vi "DMSC.manage_process.vi"(0 "Process":T1 {"restartMode" items=["UNKNOWN", "MANUAL", "ONCE", "ALWAYS", "KILL", "SHUTDOWN"]}, 1 "procNames":string[](array[string]), 2 "procID":i32[](array[numeric]), 3 "procMemory":i32[](array[numeric]), 4 "procRuntime":dbl[](array[numeric]), 5 "SDConnectionEvent":refnum<user-event>) -> (14 "Process (out)":T1 {"restartMode" items=["UNKNOWN", "MANUAL", "ONCE", "ALWAYS", "KILL", "SHUTDOWN"]})   [LabVIEW 2014, in "DMSClient.lvlib"]
doc: "Manages (start/kill) processes"
uses:
  DMSClient.lvlib
  DMSC.process_type.ctl
  DomainManagementUtils/DMSU.restart_mode.ctl
  DomainManagementUtils/DMSUtils.lvlib
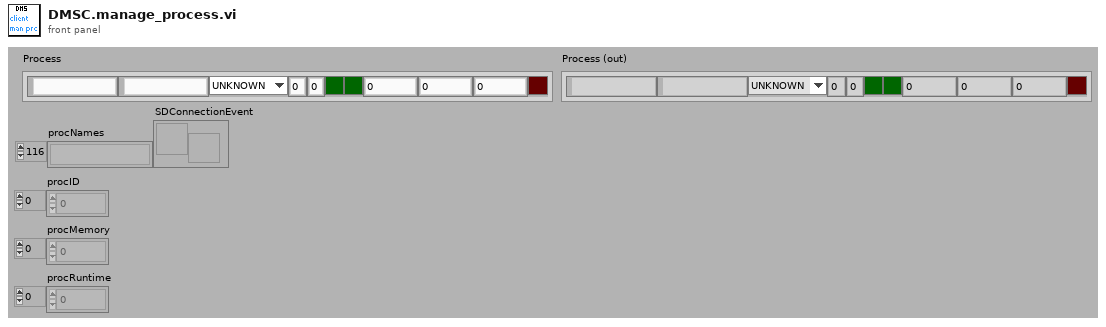
[diagram p1: front panel]
types:
  T1 = typedef "DMSClient.lvlib/DMSC.process_type.ctl" = cluster{"imageName":string, "argumentString":string, "restartMode":T2, "nOfRestart":i32, "resetRestartTimer":i32, "killOnExit":bool, "csSystem":bool, "PID":dbl, "PMem":dbl, "CPUTime":dbl, "startCnt":i32, "startTime":u32, "restartFailed":bool}
  T2 = typedef "DMSUtils.lvlib/DMSU.restart_mode.ctl" = u16
  T3 = cluster{"Command":enum16{"NewSystem", "DestroySystem", "SDSystem"}, "argumentString":string}
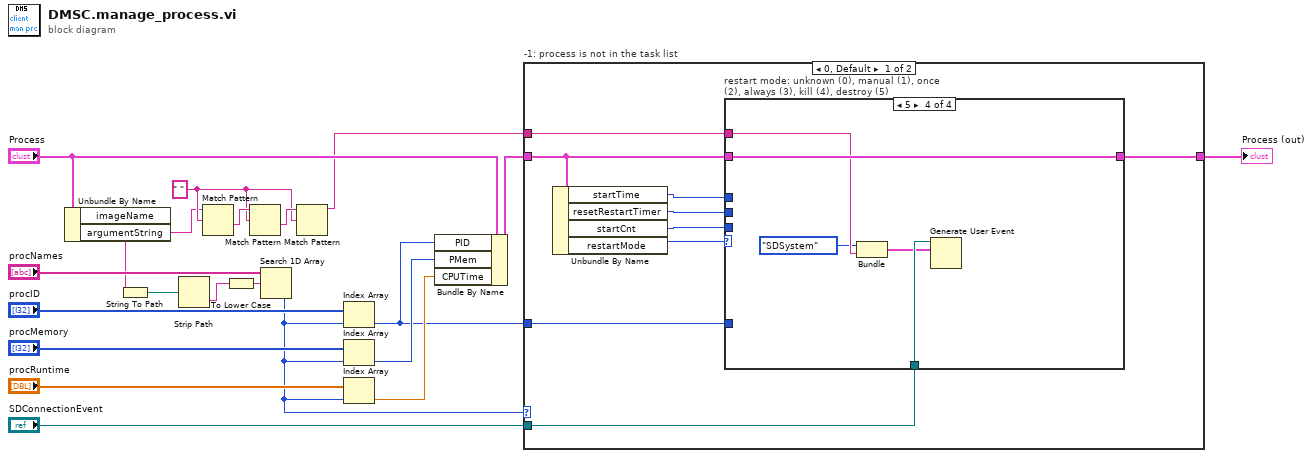
[diagram p0: block diagram]
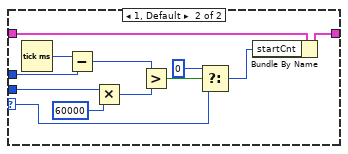
[diagram p3: hidden frame]
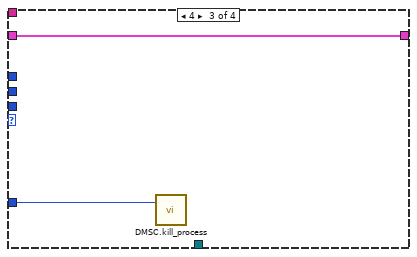
[diagram p5: hidden frame]
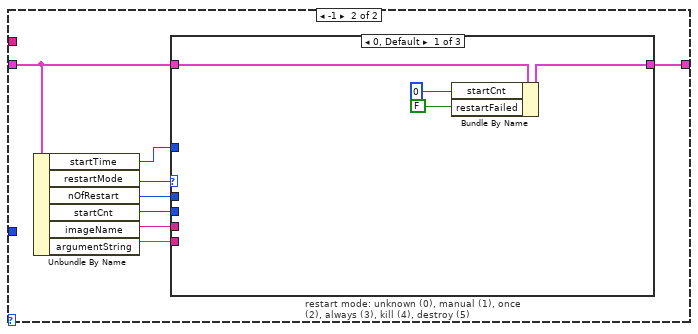
[diagram p6: hidden frame]
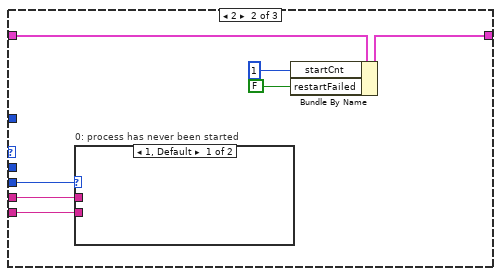
[diagram p7: hidden frame]
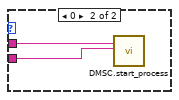
[diagram p8: hidden frame]
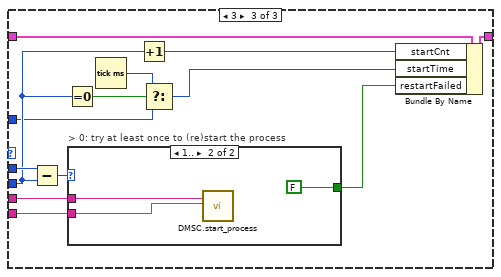
[diagram p9: hidden frame]
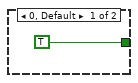
[diagram p10: hidden frame]
diagram:
  w4 = " " ("regular expression")
  n1 = Unbundle By Name("Process") -> ("imageName"=w8:string, "argumentString"=w3:string)
  n2 = String To Path(string=w8) -> (path=w9:path)
  n3 = Strip Path(path=w9) -> (name=w7:string)  [unwired: 1 out]
  n4 = Match Pattern(string=w3, regular expression=w4) -> (after substring=w6:string)  [unwired: 1 in, 3 out]
  n5 = To Lower Case(string=w7) -> (all lower case string=w10:string)
  n6 = Match Pattern(string=w6, regular expression=w4) -> (after substring=w5:string)  [unwired: 1 in, 3 out]
  n7 = Search 1D Array(1D array="procNames", element=w10) -> (index of element=w14:i32)  [unwired: 1 in]
  n8 = Match Pattern(string=w5, regular expression=w4) -> (before substring=w2:string)  [unwired: 1 in, 3 out]
  n9 = Index Array(array="procID", index=w14) -> (element=w11:i32)
  n10 = Index Array(array="procMemory", index=w14) -> (element=w21:i32)
  n11 = Index Array(array="procRuntime", index=w14) -> (element=w20:dbl)
  n12 = Bundle By Name(cluster="Process", "PID"=w11, "PMem"=w21, "CPUTime"=w20) -> (w13:T1)
  n13 = case "-1: process is not in the task list" shown="0, Default" w14 {
    tunnel: w13 -> [w28 w60]
    tunnel: [w27 w59] -> w12
    tunnel: w11 -> [w29 _]
    tunnel: w2 -> [w23 _]
    tunnel: "SDConnectionEvent" -> [w22 _]
    frame 0, Default {
      n14 = Unbundle By Name(w28) -> ("startTime"=w24:u32, "resetRestartTimer"=w25:i32, "startCnt"=w26:i32, "restartMode"=w30:T2)
      n15 = case "restart mode: unknown (0), manual (1), once (2), always (3), kill (4), destroy (5)" shown="5" w30 {
        tunnel: w29 -> [_ _ w51 _]
        tunnel: [w33 w49 w50 w56] -> w27
        tunnel: w28 -> [w34 w49 w50 w56]
        tunnel: w26 -> [w35 _ _ _]
        tunnel: w25 -> [w32 _ _ _]
        tunnel: w24 -> [w31 _ _ _]
        tunnel: w23 -> [_ _ _ w54]
        tunnel: w22 -> [_ _ _ w55]
        frame 3 {
          n16 = case "> 0: process started successfully at least once, set startCnt to 0" shown="0" w35 {
            selector: w35 -> [_ w39]
            tunnel: [w36 w37] -> w33
            tunnel: w34 -> [w36 w41]
            tunnel: w32 -> [_ w48]
            tunnel: w31 -> [_ w45]
            frame 0 {
            }
            frame 1, Default {
              n17 = Tick Count (ms)() -> (millisecond timer value=w46:u32)
              n18 = Subtract(x=w46, y=w45) -> (x-y=w44:u32)
              n19 = Multiply(x=w48, y=u32 60000) -> (x*y=w43:u32)
              n20 = Greater?(x=w44, y=w43) -> (0:w42:bool)
              n21 = Select(t=0, s=w42, f=w39) -> (s? t:f=w40:i32)
              n22 = Bundle By Name(cluster=w41, "startCnt"=w40) -> (w37:T1)
            }
          }
        }
        frame 0, Default {
        }
        frame 4 {
          n23 = call "DMSC.kill_process.vi"("PID"=w51) -> ()  [unwired: 18 in, 1 out]
        }
        frame 5 {
          n24 = Bundle("Command"=enum16{"NewSystem", "DestroySystem", "SDSystem"}."SDSystem", "argumentString"=w54) -> (w53:T3)  [unwired: 1 in]
          n25 = Generate User Event(user event=w55, event data cluster=w53) -> ()  [unwired: 2 in, 2 out]
        }
      }
    }
    frame -1 {
      n26 = Unbundle By Name(w60) -> ("startTime"=w58:u32, "restartMode"=w64:T2, "nOfRestart"=w63:i32, "startCnt"=w61:i32, "imageName"=w62:string, "argumentString"=w57:string)
      n27 = case "restart mode: unknown (0), manual (1), once (2), always (3), kill (4), destroy (5)" shown="0, Default" w64 {
        tunnel: w63 -> [_ _ w88]
        tunnel: w62 -> [_ w75 w90]
        tunnel: w57 -> [_ w74 w89]
        tunnel: w61 -> [_ w69 w83]
        tunnel: w60 -> [w68 w73 w86]
        tunnel: [w67 w72 w85] -> w59
        tunnel: w58 -> [_ _ w80]
        frame 0, Default {
          n28 = Bundle By Name(cluster=w68, "startCnt"=0, "restartFailed"=FALSE) -> (w67:T1)
        }
        frame 2 {
          n29 = case "0: process has never been started" shown="1, Default" w69 {
            tunnel: w75 -> [_ w77]
            tunnel: w74 -> [_ w76]
            frame 1, Default {
            }
            frame 0 {
              n30 = call "DMSC.start_process.vi"("imageName"=w77, "argumentString"=w76) -> ()  [unwired: 17 in, 1 out]
            }
          }
          n31 = Bundle By Name(cluster=w73, "startCnt"=1, "restartFailed"=FALSE) -> (w72:T1)
        }
        frame 3 {
          n32 = Subtract(x=w88, y=w83) -> (x-y=w87:i32)
          n33 = Equal To 0?(x=w83) -> (x = 0?=w82:bool)
          n34 = case "> 0: try at least once to (re)start the process" shown="1.." w87 {
            tunnel: w90 -> [_ w93]
            tunnel: w89 -> [_ w92]
            tunnel: [TRUE FALSE] -> w78
            frame 0, Default {
            }
            frame 1.. {
              n35 = call "DMSC.start_process.vi"("imageName"=w93, "argumentString"=w92) -> ()  [unwired: 17 in, 1 out]
            }
          }
          n36 = Tick Count (ms)() -> (millisecond timer value=w81:u32)
          n37 = Increment(x=w83) -> (x+1=w84:i32)
          n38 = Select(t=w81, s=w82, f=w80) -> (s? t:f=w79:u32)
          n39 = Bundle By Name(cluster=w86, "startCnt"=w84, "startTime"=w79, "restartFailed"=w78) -> (w85:T1)
        }
      }
    }
  }
  "Process (out)" <- w12
